vi "Number of Variables.vi"() -> (7 "Number of Variables":i32)   [LabVIEW 2015]
uses:
  variable setpoint.ctl
  data ave interval.ctl
  type specifier for control code.ctl
  logic buffer cmd.ctl
panel:
  out "Set Points out":T1[](array[typedef])=[{"name"="", "unit"="", "value"=0.0, "Type"=enum."Constant", "variable"={"selected sensors"=[], "selected set points"=[], "VI"=path "", "Data average interval"=0.0, "code ref"=refnum}}] {"value" format="%#_6p"; "variable"."Data average interval" min=0.0 format="%^#_3g"}
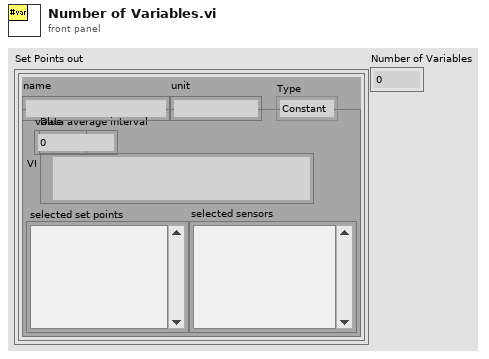
[diagram p1: front panel]
types:
  T1 = typedef "variable setpoint.ctl" = cluster{"name":string, "unit":string, "value":dbl, "Type":enum16{"Constant", "Variable"}, "variable":cluster{"selected sensors":i32[], "selected set points":i32[], "VI":path, "Data average interval":T2, "code ref":T3}}
  T2 = typedef "data ave interval.ctl" = dbl
  T3 = typedef "type specifier for control code.ctl" = refnum<vi>
  T4 = typedef "logic buffer cmd.ctl" = enum16{"read", "write ouput settings", "write rules", "write setpoints", "write output descriptions", "write all", "calculate setpoints", "save", "open", "Load all setpoint code", "Load one setpoint code", "Configure one setpoint code"}
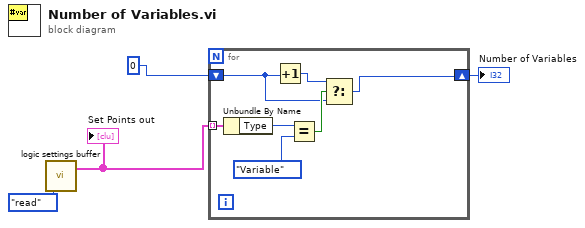
[diagram p0: block diagram]
diagram:
  n1 = call "logic settings buffer.vi"("command"=logic_buffer_cmd."read") -> ("Set Points out"=w3:T1[])  [unwired: 11 in, 7 out]
  "Set Points out" <- w3
  n2 = for {
    tunnel: w3 -> [w11] mode=indexing
    shift-right: [w7] -> w1
    shift-left: 0 -> [w5]
    n3 = Unbundle By Name(w11) -> ("Type"=w10:enum16{"Constant", "Variable"})
    n4 = Increment(x=w5) -> (x+1=w8:i32)
    n5 = Equal?(x=w10, y=enum16{"Constant", "Variable"}."Variable" ("Type")) -> (x = y?=w6:bool)
    n6 = Select(t=w8, s=w6, f=w5) -> (s? t:f=w7:i32)
  }
  "Number of Variables" <- w1
